vi "MGCC_PVFcst_main.vi"() -> ()   [LabVIEW 2016]
uses:
  Sub-VIs/f_MGCC_PVFcst_ActualPV.vi
  Finite State Machine/Sub-VIs/MGCC_FntStaMach_gobal.vi
  Communication/Global communication.vi
  Communication/Global communication output.vi
  <vilib>/Utility/error.llb/Error Cluster From Error Code.vi
  <vilib>/ErrorRing/Error Ring.xnode
  <vilib>/Analysis/NI_AALBase.lvlib
panel:
  out "f_MGCC_PVFcst_HistoricalPV 2":dbl[](graph)
  out "coerced(x) 2":dbl[](graph)
  out "f_MGCC_PVFcst_HistoricalPV":dbl[](graph)
  out "coerced(x)":dbl[](graph)
  out "error1":errorcluster
  # "Copyright <2020> <The University of Tennessee at Knoxville and the University of Tennessee Research Foundation>\n\nRedistribution and use in source and binary forms, with or without modification, are permitted provided that the following conditions are met:\n\n1. Redistributions of source code must retain the above copyright notice, this list of conditions and the following disclaimer.\n\n2. Redistributions in binary form must reproduce the above copyright notice, this list of conditions and the following disclaimer in the documentation and/or other materials provided with the distribution.\n\n3. Neither the name of the copyright holder nor the names of its contributors may be used to endorse or promote products derived from this software without specific prior written permission.\n\nTHIS SOFTWARE IS PROVIDED BY THE COPYRIGHT HOLDERS AND CONTRIBUTORS \"AS IS\" AND ANY EXPRESS OR IMPLIED WARRANTIES, INCLUDING, BUT NOT LIMITED TO, THE IMPLIED WARRANTIES OF MERCHANTABILITY AND FITNESS FOR A PARTICULAR PURPOSE ARE DISCLAIMED. IN NO EVENT SHALL THE COPYRIGHT HOLDER OR CONTRIBUTORS BE LIABLE FOR ANY DIRECT, INDIRECT, INCIDENTAL, SPECIAL, EXEMPLARY, OR CONSEQUENTIAL DAMAGES (INCLUDING, BUT NOT LIMITED TO, PROCUREMENT OF SUBSTITUTE GOODS OR SERVICES; LOSS OF USE, DATA, OR PROFITS; OR BUSINESS INTERRUPTION) HOWEVER CAUSED AND ON ANY THEORY OF LIABILITY, WHETHER IN CONTRACT, STRICT LIABILITY, OR TORT (INCLUDING NEGLIGENCE OR OTHERWISE) ARISING IN ANY WAY OUT OF THE USE OF THIS SOFTWARE, EVEN IF ADVISED OF THE POSSIBILITY OF SUCH DAMAGE."
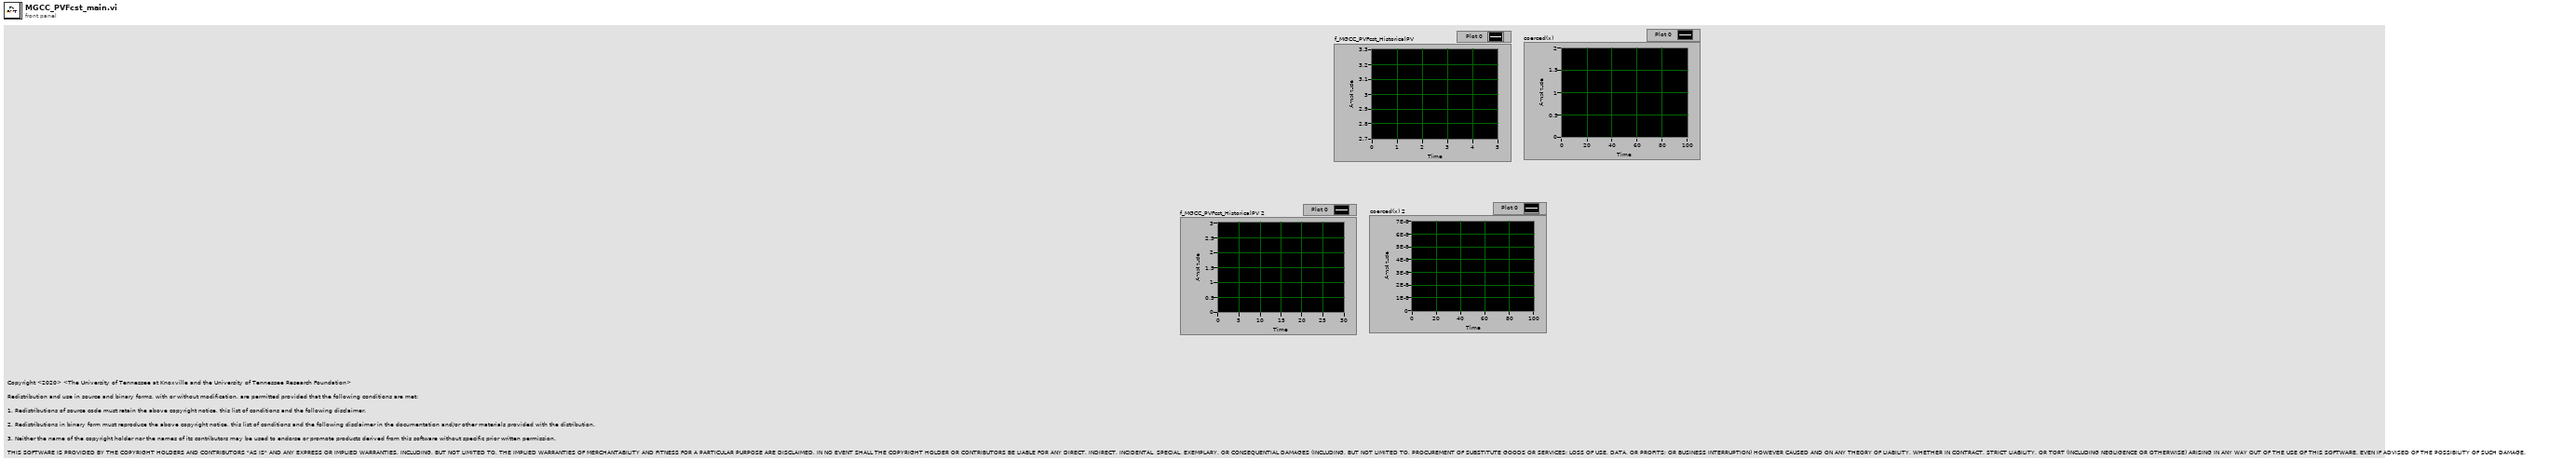
[diagram p1: front panel]
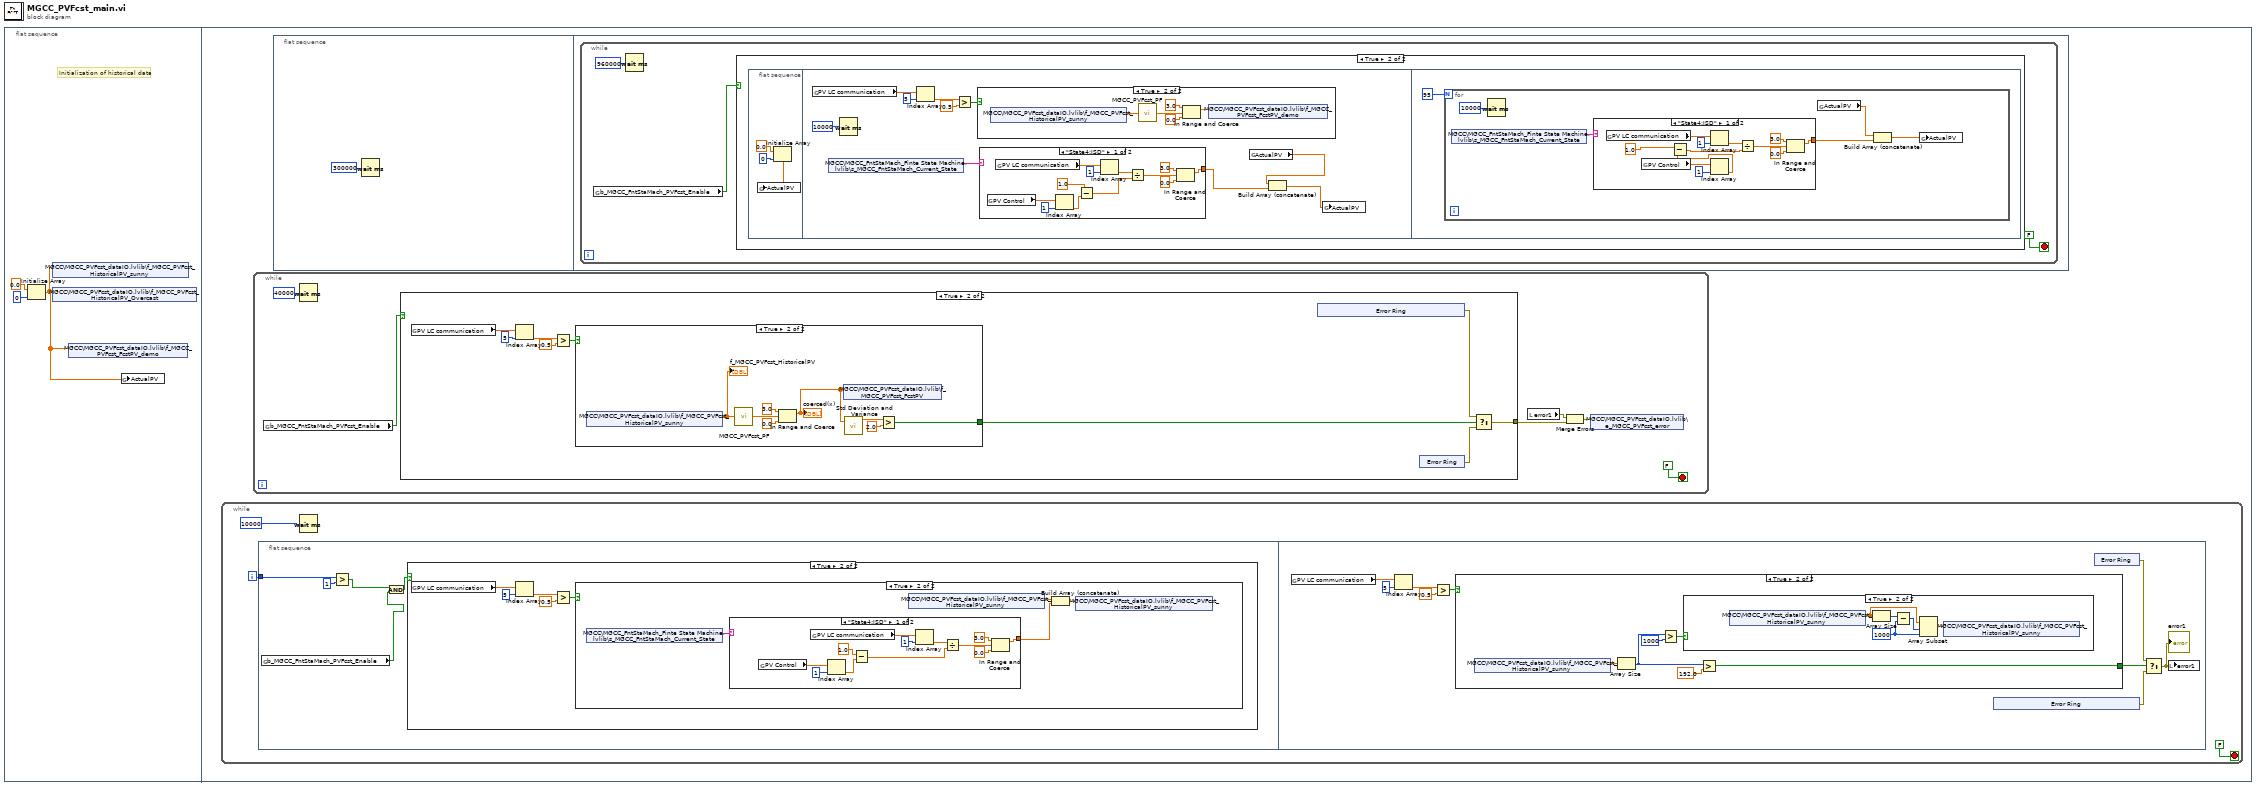
[diagram p0: block diagram]
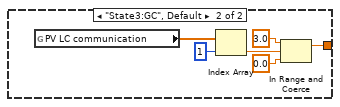
[diagram p3: hidden frame]
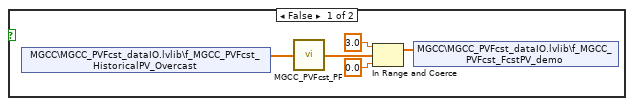
[diagram p4: hidden frame]
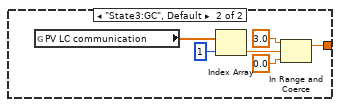
[diagram p5: hidden frame]
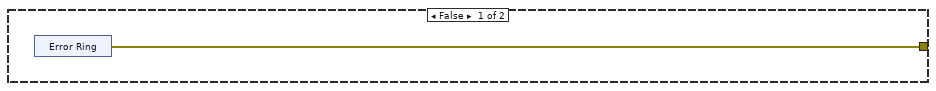
[diagram p6: hidden frame]
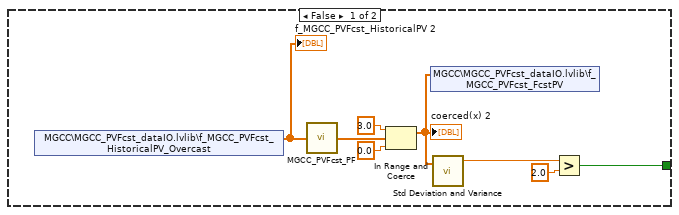
[diagram p7: hidden frame]
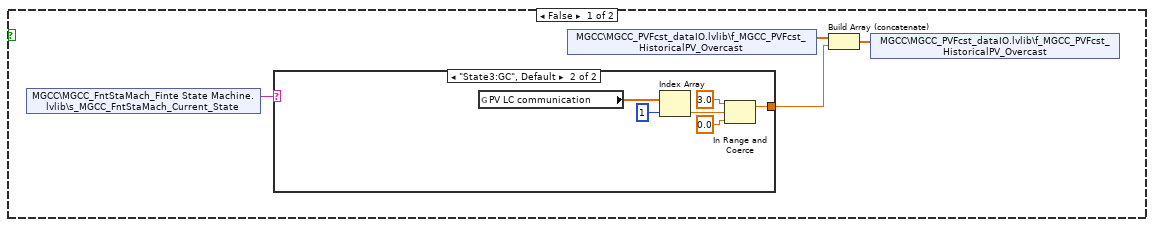
[diagram p9: hidden frame]
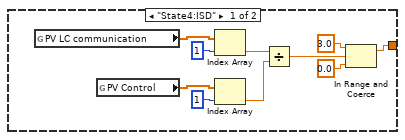
[diagram p10: hidden frame]
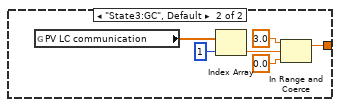
[diagram p11: hidden frame]
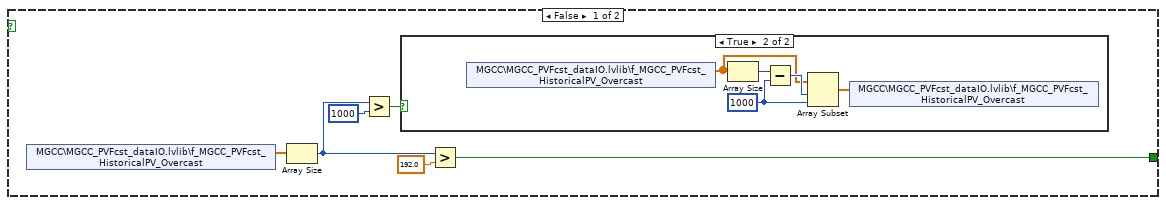
[diagram p12: hidden frame]
diagram:
  n1 = flat-sequence {
    frame #0 {
      # "Initialization of historical data"
      n2 = Initialize Array(0.0 ("element"), 0 ("dimension size")) -> (w1:dbl[])
      n3 = shared-variable "MGCC\\MGCC_PVFcst_dataIO.lvlib\\f_MGCC_PVFcst_HistoricalPV_sunny"(w1) -> ()  [unwired: 1 in, 1 out]
      n4 = shared-variable "MGCC\\MGCC_PVFcst_dataIO.lvlib\\f_MGCC_PVFcst_HistoricalPV_Overcast"(w1) -> ()  [unwired: 1 in, 1 out]
      n5 = shared-variable "MGCC\\MGCC_PVFcst_dataIO.lvlib\\f_MGCC_PVFcst_FcstPV_demo"(w1) -> ()  [unwired: 1 in, 1 out]
      n6 = global write "f_MGCC_PVFcst_ActualPV.vi" "ActualPV"(w1) -> ()
    }
    frame #1 {
      n7 = while {
        i -> [w112]
        stop <- FALSE stop-if-true
        n8 = flat-sequence {
          tunnel: w112 -> [w117]
          frame #0 {
            n9 = global read "MGCC_FntStaMach_gobal.vi" "b_MGCC_FntStaMach_PVFcst_Enable"() -> (w115:bool)
            n10 = Greater?(x=w117, y=1) -> (0:w118:bool)
            n11 = And(x=w118, y=w115) -> (x .and. y?=w116:bool)
            n12 = case shown="True" w116 {
              frame False {
              }
              frame True {
                n13 = global read "Global communication.vi" "PV LC communication"() -> (w124:dbl[])
                n14 = Index Array(array=w124, index=5) -> (element=w122:dbl)
                n15 = Greater?(x=w122, y=0.5) -> (0:w120:bool)
                n16 = case shown="True" w120 {
                  frame False {
                    n17 = shared-variable "MGCC\\MGCC_FntStaMach_Finte State Machine.lvlib\\s_MGCC_FntStaMach_Current_State"() -> (w125:string)  [unwired: 1 in, 1 out]
                    n18 = case shown="\"State3:GC\", Default" w125 {
                      tunnel: [w129 w142] -> w126
                      frame "State4:ISD" {
                        n19 = global read "Global communication.vi" "PV LC communication"() -> (w136:dbl[])
                        n20 = global read "Global communication output.vi" "PV Control"() -> (w133:dbl[])
                        n21 = Index Array(array=w136, index=1) -> (element=w130:dbl)
                        n22 = Index Array(array=w133, index=1) -> (element=w132:dbl)
                        n23 = Divide(x=w130, y=w132) -> (x/y=w131:dbl)
                        n24 = In Range and Coerce(upper limit=3.0, x=w131, lower limit=0.0) -> (coerced(x)=w129:dbl)  [unwired: 1 out]
                      }
                      frame "State3:GC", Default {
                        n25 = global read "Global communication.vi" "PV LC communication"() -> (w141:dbl[])
                        n26 = Index Array(array=w141, index=1) -> (element=w139:dbl)
                        n27 = In Range and Coerce(upper limit=3.0, x=w139, lower limit=0.0) -> (coerced(x)=w142:dbl)  [unwired: 1 out]
                      }
                    }
                    n28 = shared-variable "MGCC\\MGCC_PVFcst_dataIO.lvlib\\f_MGCC_PVFcst_HistoricalPV_Overcast"() -> (w128:dbl[])  [unwired: 1 in, 1 out]
                    n29 = Build Array (concatenate)(w128, w126) -> (w127:dbl[])
                    n30 = shared-variable "MGCC\\MGCC_PVFcst_dataIO.lvlib\\f_MGCC_PVFcst_HistoricalPV_Overcast"(w127) -> ()  [unwired: 1 in, 1 out]
                  }
                  frame True {
                    n31 = shared-variable "MGCC\\MGCC_FntStaMach_Finte State Machine.lvlib\\s_MGCC_FntStaMach_Current_State"() -> (w146:string)  [unwired: 1 in, 1 out]
                    n32 = case shown="\"State4:ISD\"" w146 {
                      tunnel: [w152 w164] -> w145
                      frame "State4:ISD" {
                        n33 = global read "Global communication output.vi" "PV Control"() -> (w155:dbl[])
                        n34 = global read "Global communication.vi" "PV LC communication"() -> (w158:dbl[])
                        n35 = Index Array(array=w155, index=1) -> (element=w151:dbl)
                        n36 = Subtract(x=1.0, y=w151) -> (x-y=w149:dbl)
                        n37 = Index Array(array=w158, index=1) -> (element=w153:dbl)
                        n38 = Divide(x=w153, y=w149) -> (x/y=w154:dbl)
                        n39 = In Range and Coerce(upper limit=3.0, x=w154, lower limit=0.0) -> (coerced(x)=w152:dbl)  [unwired: 1 out]
                      }
                      frame "State3:GC", Default {
                        n40 = global read "Global communication.vi" "PV LC communication"() -> (w163:dbl[])
                        n41 = Index Array(array=w163, index=1) -> (element=w161:dbl)
                        n42 = In Range and Coerce(upper limit=3.0, x=w161, lower limit=0.0) -> (coerced(x)=w164:dbl)  [unwired: 1 out]
                      }
                    }
                    n43 = shared-variable "MGCC\\MGCC_PVFcst_dataIO.lvlib\\f_MGCC_PVFcst_HistoricalPV_sunny"() -> (w148:dbl[])  [unwired: 1 in, 1 out]
                    n44 = Build Array (concatenate)(w148, w145) -> (w147:dbl[])
                    n45 = shared-variable "MGCC\\MGCC_PVFcst_dataIO.lvlib\\f_MGCC_PVFcst_HistoricalPV_sunny"(w147) -> ()  [unwired: 1 in, 1 out]
                  }
                }
              }
            }
          }
          frame #1 {
            n46 = global read "Global communication.vi" "PV LC communication"() -> (w171:dbl[])
            n47 = Index Array(array=w171, index=5) -> (element=w169:dbl)
            n48 = Greater?(x=w169, y=0.5) -> (0:w167:bool)
            n49 = case shown="True" w167 {
              tunnel: [w177 w187] -> w173
              frame False {
                n50 = shared-variable "MGCC\\MGCC_PVFcst_dataIO.lvlib\\f_MGCC_PVFcst_HistoricalPV_Overcast"() -> (w178:dbl[])  [unwired: 1 in, 1 out]
                n51 = Array Size(array=w178) -> (size(s)=w181:i32)
                n52 = Greater?(x=w181, y=1000) -> (0:w176:bool)
                n53 = case shown="True" w176 {
                  frame False {
                  }
                  frame True {
                    w186 = 1000 ("y")
                    n54 = shared-variable "MGCC\\MGCC_PVFcst_dataIO.lvlib\\f_MGCC_PVFcst_HistoricalPV_Overcast"() -> (w182:dbl[])  [unwired: 1 in, 1 out]
                    n55 = Array Size(array=w182) -> (size(s)=w183:i32)
                    n56 = Subtract(x=w183, y=w186) -> (x-y=w184:i32)
                    n57 = Array Subset(array=w182, index=w184, length=w186) -> (w185:dbl[])
                    n58 = shared-variable "MGCC\\MGCC_PVFcst_dataIO.lvlib\\f_MGCC_PVFcst_HistoricalPV_Overcast"(w185) -> ()  [unwired: 1 in, 1 out]
                  }
                }
                n59 = Greater?(x=w181, y=192.0) -> (0:w177:bool)
              }
              frame True {
                n60 = shared-variable "MGCC\\MGCC_PVFcst_dataIO.lvlib\\f_MGCC_PVFcst_HistoricalPV_sunny"() -> (w192:dbl[])  [unwired: 1 in, 1 out]
                n61 = Array Size(array=w192) -> (size(s)=w188:i32)
                n62 = Greater?(x=w188, y=1000) -> (0:w190:bool)
                n63 = case shown="True" w190 {
                  frame False {
                  }
                  frame True {
                    w193 = 1000 ("y")
                    n64 = shared-variable "MGCC\\MGCC_PVFcst_dataIO.lvlib\\f_MGCC_PVFcst_HistoricalPV_sunny"() -> (w197:dbl[])  [unwired: 1 in, 1 out]
                    n65 = Array Size(array=w197) -> (size(s)=w196:i32)
                    n66 = Subtract(x=w196, y=w193) -> (x-y=w195:i32)
                    n67 = Array Subset(array=w197, index=w195, length=w193) -> (w194:dbl[])
                    n68 = shared-variable "MGCC\\MGCC_PVFcst_dataIO.lvlib\\f_MGCC_PVFcst_HistoricalPV_sunny"(w194) -> ()  [unwired: 1 in, 1 out]
                  }
                }
                n69 = Greater?(x=w188, y=192.0) -> (0:w187:bool)
              }
            }
            n70 = xnode "Error Ring"() -> ("error out"=w174:errorcluster)
            n71 = xnode "Error Ring"() -> ("error out"=w175:errorcluster)
            n72 = Select(t=w175, s=w173, f=w174) -> (s? t:f=w172:errorcluster)
            "error1" <- w172
            n73 = local write "error1"(w172) -> ()
          }
        }
        n74 = Wait (ms)(milliseconds to wait=u32 10000) -> ()  [unwired: 1 out]
      }
      n75 = while {
        stop <- FALSE stop-if-true
        n76 = global read "MGCC_FntStaMach_gobal.vi" "b_MGCC_FntStaMach_PVFcst_Enable"() -> (w73:bool)
        n77 = Wait (ms)(milliseconds to wait=u32 40000) -> ()  [unwired: 1 out]
        n78 = case shown="True" w73 {
          tunnel: [w79 w86] -> w76
          frame False {
            n79 = xnode "Error Ring"() -> ("error out"=w79:errorcluster)
          }
          frame True {
            n80 = global read "Global communication.vi" "PV LC communication"() -> (w85:dbl[])
            n81 = Index Array(array=w85, index=5) -> (element=w83:dbl)
            n82 = Greater?(x=w83, y=0.5) -> (0:w81:bool)
            n83 = case shown="True" w81 {
              tunnel: [w90 w99] -> w87
              frame False {
                n84 = shared-variable "MGCC\\MGCC_PVFcst_dataIO.lvlib\\f_MGCC_PVFcst_HistoricalPV_Overcast"() -> (w91:dbl[])  [unwired: 1 in, 1 out]
                "f_MGCC_PVFcst_HistoricalPV 2" <- w91
                n85 = call "MGCC_PVFcst_PF.vi"("InputTimeSeries"=w91) -> ("predicted series"=w94:dbl[])
                n86 = In Range and Coerce(upper limit=3.0, x=w94, lower limit=0.0) -> (coerced(x)=w97:dbl[])  [unwired: 1 out]
                "coerced(x) 2" <- w97
                n87 = shared-variable "MGCC\\MGCC_PVFcst_dataIO.lvlib\\f_MGCC_PVFcst_FcstPV"(w97) -> ()  [unwired: 1 in, 1 out]
                n88 = call <vilib>:"Std Deviation and Variance.vi"("X"=w97) -> ("mean"=w96:dbl)  [unwired: 1 in, 2 out]
                n89 = Greater?(x=w96, y=2.0) -> (0:w90:bool)
              }
              frame True {
                n90 = shared-variable "MGCC\\MGCC_PVFcst_dataIO.lvlib\\f_MGCC_PVFcst_HistoricalPV_sunny"() -> (w105:dbl[])  [unwired: 1 in, 1 out]
                "f_MGCC_PVFcst_HistoricalPV" <- w105
                n91 = call "MGCC_PVFcst_PF.vi"("InputTimeSeries"=w105) -> ("predicted series"=w103:dbl[])
                n92 = In Range and Coerce(upper limit=3.0, x=w103, lower limit=0.0) -> (coerced(x)=w100:dbl[])  [unwired: 1 out]
                "coerced(x)" <- w100
                n93 = shared-variable "MGCC\\MGCC_PVFcst_dataIO.lvlib\\f_MGCC_PVFcst_FcstPV"(w100) -> ()  [unwired: 1 in, 1 out]
                n94 = call <vilib>:"Std Deviation and Variance.vi"("X"=w100) -> ("mean"=w101:dbl)  [unwired: 1 in, 2 out]
                n95 = Greater?(x=w101, y=2.0) -> (0:w99:bool)
              }
            }
            n96 = xnode "Error Ring"() -> ("error out"=w89:errorcluster)
            n97 = xnode "Error Ring"() -> ("error out"=w88:errorcluster)
            n98 = Select(t=w89, s=w87, f=w88) -> (s? t:f=w86:errorcluster)
          }
        }
        n99 = local read "error1"() -> (w74:errorcluster)
        n100 = Merge Errors(w74, w76) -> (w75:errorcluster)
        n101 = shared-variable "MGCC\\MGCC_PVFcst_dataIO.lvlib\\e_MGCC_PVFcst_error"(w75) -> ()  [unwired: 1 in, 1 out]
      }
      n102 = flat-sequence {
        frame #0 {
          n103 = Wait (ms)(milliseconds to wait=u32 300000) -> ()  [unwired: 1 out]
        }
        frame #1 {
          n104 = while {
            stop <- FALSE stop-if-true
            n105 = global read "MGCC_FntStaMach_gobal.vi" "b_MGCC_FntStaMach_PVFcst_Enable"() -> (w5:bool)
            n106 = Wait (ms)(milliseconds to wait=u32 960000) -> ()  [unwired: 1 out]
            n107 = case shown="True" w5 {
              frame False {
              }
              frame True {
                n108 = flat-sequence {
                  frame #0 {
                    n109 = Initialize Array(0.0 ("element"), 0 ("dimension size")) -> (w10:dbl[])
                    n110 = global write "f_MGCC_PVFcst_ActualPV.vi" "ActualPV"(w10) -> ()
                  }
                  frame #1 {
                    n111 = global read "Global communication.vi" "PV LC communication"() -> (w20:dbl[])
                    n112 = shared-variable "MGCC\\MGCC_FntStaMach_Finte State Machine.lvlib\\s_MGCC_FntStaMach_Current_State"() -> (w15:string)  [unwired: 1 in, 1 out]
                    n113 = Wait (ms)(milliseconds to wait=u32 10000) -> ()  [unwired: 1 out]
                    n114 = Index Array(array=w20, index=5) -> (element=w18:dbl)
                    n115 = Greater?(x=w18, y=0.5) -> (0:w16:bool)
                    n116 = case shown="True" w16 {
                      frame False {
                        n117 = shared-variable "MGCC\\MGCC_PVFcst_dataIO.lvlib\\f_MGCC_PVFcst_HistoricalPV_Overcast"() -> (w39:dbl[])  [unwired: 1 in, 1 out]
                        n118 = call "MGCC_PVFcst_PF.vi"("InputTimeSeries"=w39) -> ("predicted series"=w42:dbl[])
                        n119 = In Range and Coerce(upper limit=3.0, x=w42, lower limit=0.0) -> (coerced(x)=w43:dbl[])  [unwired: 1 out]
                        n120 = shared-variable "MGCC\\MGCC_PVFcst_dataIO.lvlib\\f_MGCC_PVFcst_FcstPV_demo"(w43) -> ()  [unwired: 1 in, 1 out]
                      }
                      frame True {
                        n121 = shared-variable "MGCC\\MGCC_PVFcst_dataIO.lvlib\\f_MGCC_PVFcst_HistoricalPV_sunny"() -> (w48:dbl[])  [unwired: 1 in, 1 out]
                        n122 = call "MGCC_PVFcst_PF.vi"("InputTimeSeries"=w48) -> ("predicted series"=w45:dbl[])
                        n123 = In Range and Coerce(upper limit=3.0, x=w45, lower limit=0.0) -> (coerced(x)=w44:dbl[])  [unwired: 1 out]
                        n124 = shared-variable "MGCC\\MGCC_PVFcst_dataIO.lvlib\\f_MGCC_PVFcst_FcstPV_demo"(w44) -> ()  [unwired: 1 in, 1 out]
                      }
                    }
                    n125 = case shown="\"State4:ISD\"" w15 {
                      tunnel: [w24 w36] -> w13
                      frame "State4:ISD" {
                        n126 = global read "Global communication output.vi" "PV Control"() -> (w27:dbl[])
                        n127 = global read "Global communication.vi" "PV LC communication"() -> (w30:dbl[])
                        n128 = Index Array(array=w27, index=1) -> (element=w23:dbl)
                        n129 = Subtract(x=1.0, y=w23) -> (x-y=w21:dbl)
                        n130 = Index Array(array=w30, index=1) -> (element=w25:dbl)
                        n131 = Divide(x=w25, y=w21) -> (x/y=w26:dbl)
                        n132 = In Range and Coerce(upper limit=3.0, x=w26, lower limit=0.0) -> (coerced(x)=w24:dbl)  [unwired: 1 out]
                      }
                      frame "State3:GC", Default {
                        n133 = global read "Global communication.vi" "PV LC communication"() -> (w35:dbl[])
                        n134 = Index Array(array=w35, index=1) -> (element=w33:dbl)
                        n135 = In Range and Coerce(upper limit=3.0, x=w33, lower limit=0.0) -> (coerced(x)=w36:dbl)  [unwired: 1 out]
                      }
                    }
                    n136 = global read "f_MGCC_PVFcst_ActualPV.vi" "ActualPV"() -> (w12:dbl[])
                    n137 = Build Array (concatenate)(w12, w13) -> (w11:dbl[])
                    n138 = global write "f_MGCC_PVFcst_ActualPV.vi" "ActualPV"(w11) -> ()
                  }
                  frame #2 {
                    n139 = for {
                      N: 95 -> [_]
                      n140 = shared-variable "MGCC\\MGCC_FntStaMach_Finte State Machine.lvlib\\s_MGCC_FntStaMach_Current_State"() -> (w53:string)  [unwired: 1 in, 1 out]
                      n141 = Wait (ms)(milliseconds to wait=u32 10000) -> ()  [unwired: 1 out]
                      n142 = case shown="\"State4:ISD\"" w53 {
                        tunnel: [w58 w70] -> w52
                        frame "State4:ISD" {
                          n143 = global read "Global communication.vi" "PV LC communication"() -> (w64:dbl[])
                          n144 = global read "Global communication output.vi" "PV Control"() -> (w61:dbl[])
                          n145 = Index Array(array=w64, index=1) -> (element=w59:dbl)
                          n146 = Index Array(array=w61, index=1) -> (element=w56:dbl)
                          n147 = Subtract(x=1.0, y=w56) -> (x-y=w55:dbl)
                          n148 = Divide(x=w59, y=w55) -> (x/y=w60:dbl)
                          n149 = In Range and Coerce(upper limit=3.0, x=w60, lower limit=0.0) -> (coerced(x)=w58:dbl)  [unwired: 1 out]
                        }
                        frame "State3:GC", Default {
                          n150 = global read "Global communication.vi" "PV LC communication"() -> (w69:dbl[])
                          n151 = Index Array(array=w69, index=1) -> (element=w67:dbl)
                          n152 = In Range and Coerce(upper limit=3.0, x=w67, lower limit=0.0) -> (coerced(x)=w70:dbl)  [unwired: 1 out]
                        }
                      }
                      n153 = global read "f_MGCC_PVFcst_ActualPV.vi" "ActualPV"() -> (w50:dbl[])
                      n154 = Build Array (concatenate)(w50, w52) -> (w51:dbl[])
                      n155 = global write "f_MGCC_PVFcst_ActualPV.vi" "ActualPV"(w51) -> ()
                    }
                  }
                }
              }
            }
          }
        }
      }
    }
  }
